vi "AD得到最大误差.vi"(8 "第几组":i32, 10 "新误差值":dbl) -> ()   [LabVIEW 2010]
uses:
  全局量/自动测试结果.vi
panel:
  # "从0开始"
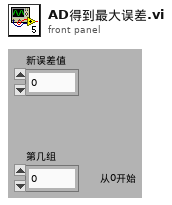
[diagram p1: front panel]
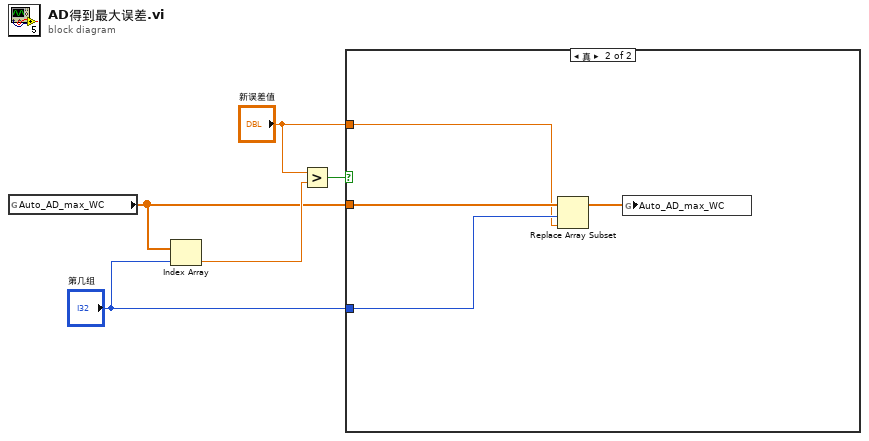
[diagram p0: block diagram]
diagram:
  n1 = global read "自动测试结果.vi" "Auto_AD_max_WC"() -> (w3:dbl[])
  n2 = Index Array(array=w3, index="第几组") -> (element=w5:dbl)
  n3 = Greater?(x="新误差值", y=w5) -> (0:w4:bool)
  n4 = case shown="真" w4 {
    tunnel: w3 -> [_ w9]
    tunnel: "第几组" -> [_ w7]
    tunnel: "新误差值" -> [_ w6]
    frame False {
    }
    frame True {
      n5 = Replace Array Subset(array=w9, new element=w6, index=w7) -> (w8:dbl[])
      n6 = global write "自动测试结果.vi" "Auto_AD_max_WC"(w8) -> ()
    }
  }
